vi "DM get group info.vi"(10 "group":string, 11 "module loopdata in":T1) -> (2 "group info":T3, 3 "module loopdata out":T1)   [LabVIEW 2019, in "DataManagment.lvlib"]
uses:
  DataManagment.lvlib
  DM group info.ctl
  module data.ctl
  SubVIs/mmWave data_class/mmWave data.lvclass
  DM signal group.ctl
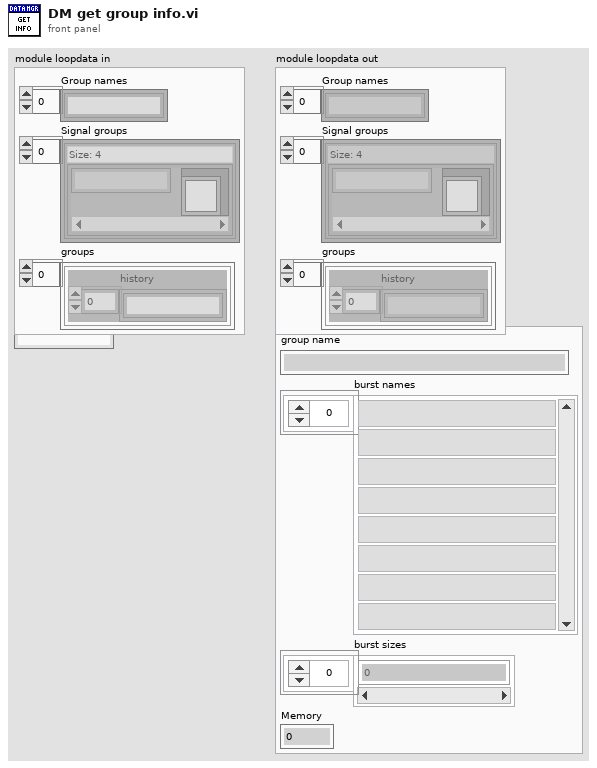
[diagram p1: front panel]
types:
  T1 = typedef "DataManagment.lvlib/module data.ctl" = cluster{"Group names":string[], "Signal groups":map{string, refnum<class "mmWave data.lvclass">}[], "groups":T2[]}
  T2 = typedef "DataManagment.lvlib/DM signal group.ctl" = cluster{"history":string[]}
  T3 = typedef "DataManagment.lvlib/DM group info.ctl" = cluster{"group name":string, "burst names":string[], "burst sizes":dbl[], "Memory":dbl}
  T4 = map{string, refnum<class "mmWave data.lvclass">}[]
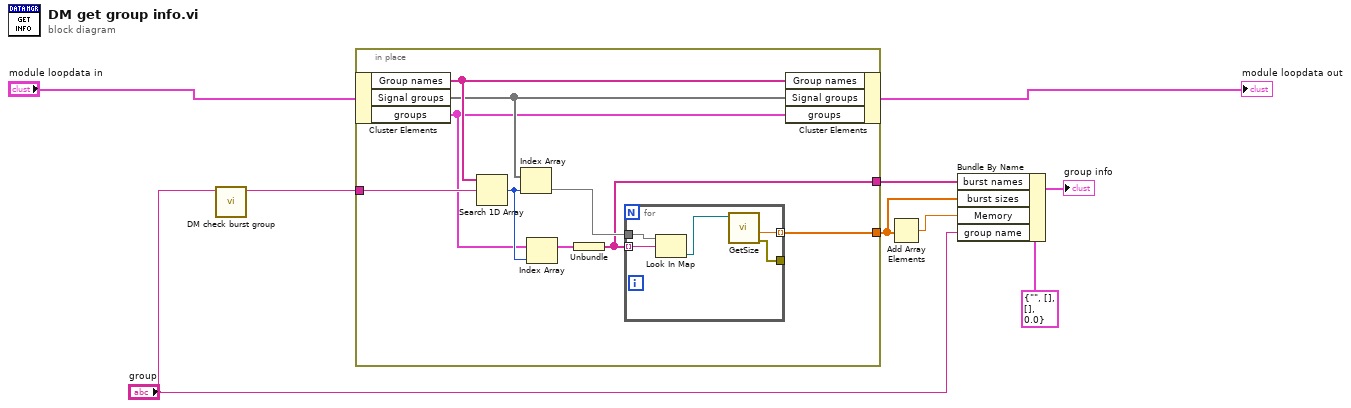
[diagram p0: block diagram]
diagram:
  n1 = call "DM check burst group.vi"("group"="group") -> ("String"=w7:string)  [unwired: 10 in]
  n2 = in-place {
    in-place-border: w7 -> [w15]
    in-place-border: [w14] -> w9
    in-place-border: [w11] -> w1
    n3 = in-place-cluster #1("module loopdata in") -> ("Group names"=w18:string[], "Signal groups"=w17:T4, "groups"=w10:T2[])
    n4 = Search 1D Array(1D array=w18, element=w15) -> (index of element=w12:i32)  [unwired: 1 in]
    n5 = Index Array(array=w17, index=w12) -> (element=w16:map{string, refnum<class "mmWave data.lvclass">})
    n6 = Index Array(array=w10, index=w12) -> (element=w13:T2)
    n7 = Unbundle(w13) -> ("history"=w11:string[])
    n8 = for {
      tunnel: w16 -> [w21]
      tunnel: [w23] -> w14 mode=indexing
      tunnel: w11 -> [w22] mode=indexing
      tunnel: [w19] -> _
      n9 = Look In Map(map=w21, key=w22) -> (value=w20:refnum<class "mmWave data.lvclass">)  [unwired: 1 in, 1 out]
      n10 = call-dynamic "GetSize.vi"("reference in"=w20) -> ("error out"=w19:errorcluster, "Size (Bytes)"=w23:dbl)  [unwired: 7 in, 2 out]
    }
    n11 = in-place-cluster #1("Group names"=w18, "Signal groups"=w17, "groups"=w10) -> (→"module loopdata out":T1)
  }
  n12 = Add Array Elements(numeric array=w9) -> (sum=w8:dbl)
  n13 = Bundle By Name(cluster=T3 {"group name"="", "burst names"=[], "burst sizes"=[], "Memory"=0.0} ("group info"), "burst names"=w1, "burst sizes"=w9, "Memory"=w8, "group name"="group") -> (→"group info":T3)
